vi "Plot Y-axis visibility.vi"(7 "Force update? (F)":bool, 8 "error in (no error)":errorcluster, 10 "top array":T1[](array[typedef]), 11 "Refs":T2) -> (0 "error out":errorcluster)   [LabVIEW 2021, in "RocketPlot.lvlib"]
uses:
  RocketPlot.lvlib
  TypeDefs/Plot UI references.ctl
  Classes/RocketPlotHandle/RocketPlotHandle.lvclass
  <userlib>/bjustice/TipStripOOPanel/Classes/TipPanelHandle/TipPanelHandle.lvclass
  TypeDefs/Plot top row.ctl
  Plot scale refnum to LUT name.vi
  FormatStringTime.vi
  Plot AxisFocus position.vi
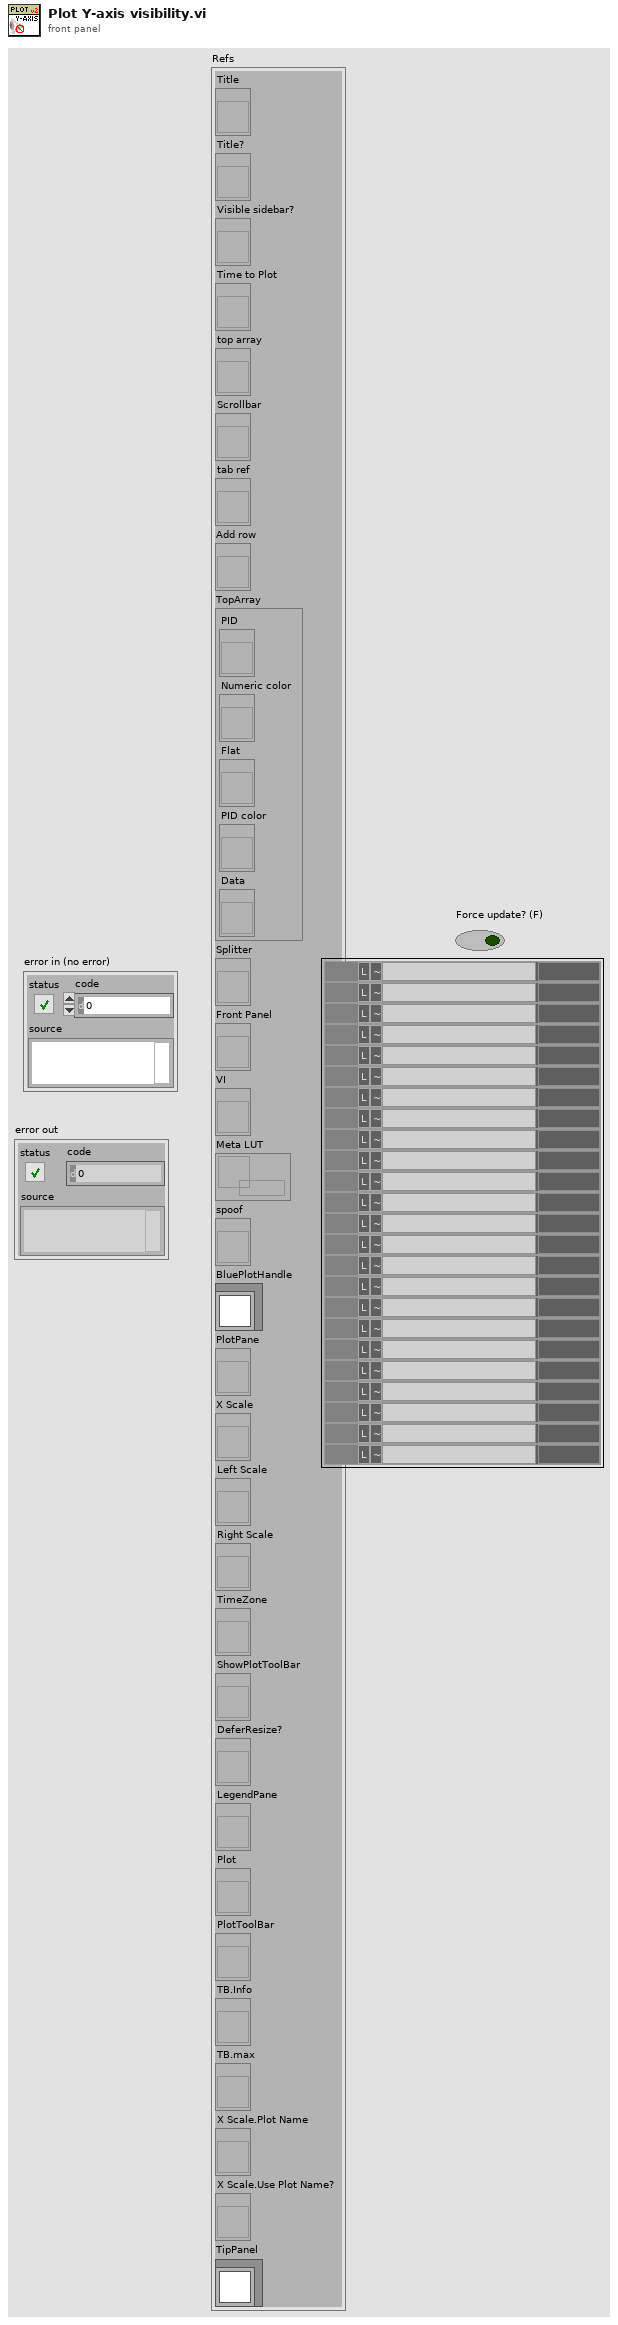
[diagram p1: front panel]
types:
  T1 = typedef "RocketPlot.lvlib/Plot top row.ctl" = cluster{"PID":string, "index":i32, "PID color":u32, "right axis?":bool, "Flatline?":bool, "Numeric color":u32, "Data":string, "Flat":string}
  T2 = typedef "RocketPlot.lvlib/Plot UI references.ctl" = cluster{"Title":refnum<vi>, "Title?":refnum<vi>, "Visible sidebar?":refnum<vi>, "Time to Plot":refnum<vi>, "top array":refnum<vi>, "Scrollbar":refnum<vi>, "tab ref":refnum<vi>, "Add row":refnum<vi>, "TopArray":cluster{"PID":refnum<vi>, "Numeric color":refnum<vi>, "Flat":refnum<vi>, "PID color":refnum<vi>, "Data":refnum<vi>}, "Splitter":refnum<vi>, "Front Panel":refnum<vi>, "VI":refnum<vi>, "Meta LUT":refnum<data-value>, "spoof":refnum<vi>, "BluePlotHandle":refnum<class "RocketPlotHandle.lvclass">, "PlotPane":refnum<vi>, "X Scale":refnum<vi>, "Left Scale":refnum<vi>, "Right Scale":refnum<vi>, "TimeZone":refnum<vi>, "ShowPlotToolBar":refnum<vi>, "DeferResize?":refnum<vi>, "LegendPane":refnum<vi>, "Plot":refnum<vi>, "PlotToolBar":refnum<vi>, "TB.Info":refnum<vi>, "TB.max":refnum<vi>, "X Scale.Plot Name":refnum<vi>, "X Scale.Use Plot Name?":refnum<vi>, "TipPanel":refnum<class "TipPanelHandle.lvclass">}
  T3 = typedef "TimeZone.ctl" = enum16{"UTC", "Local"}
  T4 = typedef "RocketPlot.lvlib/Plot scale meta JSON.ctl" = cluster{"Type":T5, "Grid Colors:Major Color":u32, "Grid Colors:Minor Color":u32, "Style":u8, "Tick Colors:Tick Color":u32, "Tick Colors:Minor Tick Color":u32, "Format String":string, "State":T6, "AxisFocus":refnum<vi>}
  T5 = typedef "RocketPlot.lvlib/Plot axis.ctl" = enum16{"x axis", "left axis", "right axis"}
  T6 = typedef "RocketPlot.lvlib/Plot scale meta state.ctl" = cluster{"Visible":bool, "Focus":bool, "Multi-Y":bool}
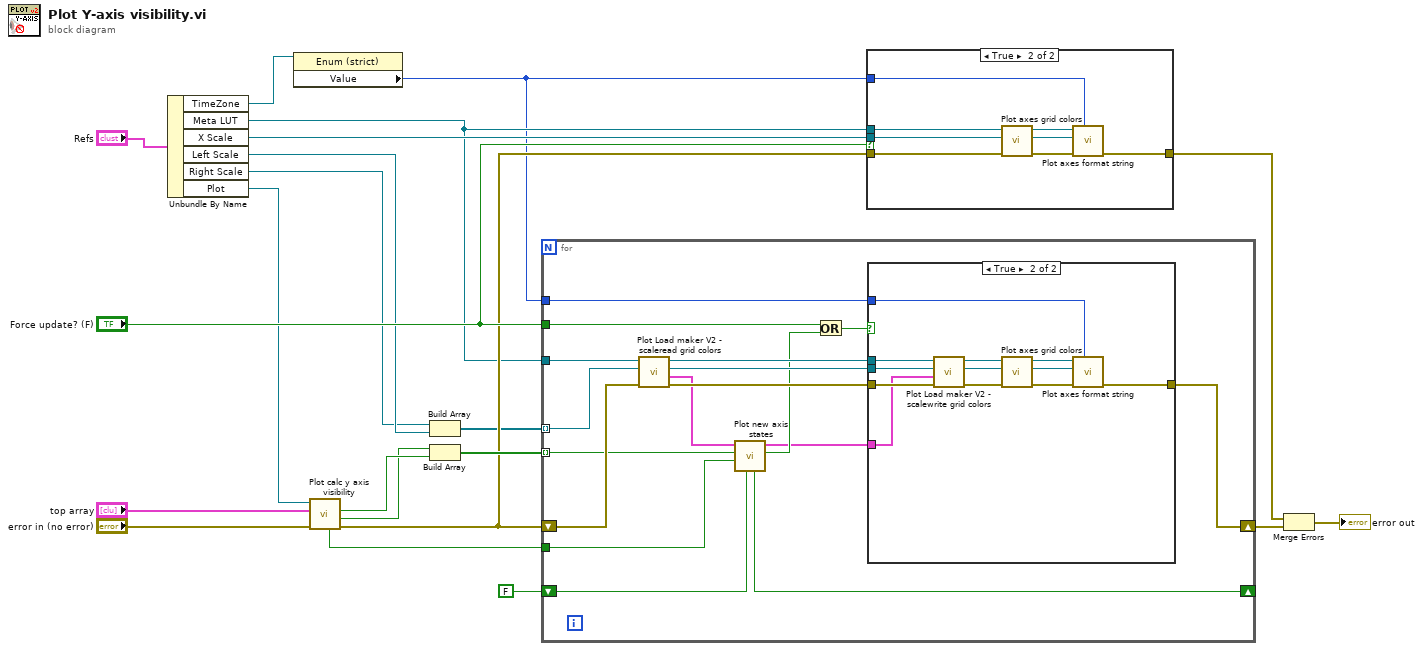
[diagram p0: block diagram]
diagram:
  n1 = Unbundle By Name("Refs") -> ("TimeZone"=w15:refnum<vi>, "Meta LUT"=w6:refnum<data-value>, "X Scale"=w8:refnum<vi>, "Left Scale"=w11:refnum<vi>, "Right Scale"=w10:refnum<vi>, "Plot"=w7:refnum<vi>)
  n2 = property class="Enum (strict)"(reference=w15) -> ("Value"=w5:T3)  [unwired: 1 in, 2 out]
  n3 = call "Plot calc y axis visibility.vi"("error in (no error)"="error in (no error)", "top array"="top array", "Plot"=w7) -> ("error out"=w14:errorcluster, "Right axis visible?"=w12:bool, "Left axis visible?"=w13:bool, "Multi-Y?"=w4:bool)  [unwired: 4 in, 1 out]
  n4 = Build Array(w10, w11) -> (w9:refnum<vi>[])
  n5 = Build Array(w12, w13) -> (w21:bool[])
  n6 = for {
    shift-right: [w38] -> w20
    shift-left: w14 -> [w32]
    tunnel: w21 -> [w26] mode=indexing
    tunnel: w6 -> [w37]
    tunnel: "Force update? (F)" -> [w30]
    tunnel: w9 -> [w33] mode=indexing
    tunnel: w5 -> [w31]
    tunnel: w4 -> [w25]
    shift-right: [w22] -> _
    shift-left: FALSE ("Multi-Y?") -> [w23]
    n7 = call "Plot Load maker V2 - scaleread grid colors.vi"("error in (no error)"=w32, "Scale reference"=w33, "Meta LUT"=w37) -> ("error out"=w34:errorcluster, "Scale LUT meta"=w28:T4, "Scale reference"=w36:refnum<vi>, "Meta LUT"=w35:refnum<data-value>)  [unwired: 5 in]
    n8 = call "Plot new axis states.vi"("GiveFocus?"=w23, "Multi-Y?"=w25, "Visible"=w26, "Scale LUT meta"=w28) -> ("state change?"=w27:bool, "Scale LUT meta"=w24:T4, "Multi-y & no-focus"=w22:bool)  [unwired: 5 in]
    n9 = Or(x=w30, y=w27) -> (x .or. y?=w29:bool)
    n10 = case shown="True" w29 {
      tunnel: [w39 w44] -> w38
      tunnel: w36 -> [_ w51]
      tunnel: w35 -> [_ w50]
      tunnel: w34 -> [w39 w49]
      tunnel: w31 -> [_ w40]
      tunnel: w24 -> [_ w41]
      frame False {
      }
      frame True {
        n11 = call "Plot Load maker V2 - scalewrite grid colors.vi"("error in (no error)"=w49, "Meta"=w41, "Scale reference"=w51, "Meta LUT"=w50) -> ("error out"=w47:errorcluster, "Scale reference"=w48:refnum<vi>, "Meta LUT"=w46:refnum<data-value>)  [unwired: 5 in]
        n12 = call "Plot axes grid colors.vi"("error in (no error)"=w47, "Scale reference"=w48, "Meta LUT"=w46) -> ("error out"=w45:errorcluster, "Scale reference"=w42:refnum<vi>, "Meta LUT"=w43:refnum<data-value>)  [unwired: 6 in]
        n13 = call "Plot axes format string.vi"("TimeZone"=w40, "error in (no error)"=w45, "Scale reference"=w42, "Meta LUT"=w43) -> ("error out"=w44:errorcluster)  [unwired: 6 in, 1 out]
      }
    }
  }
  n14 = case shown="True" "Force update? (F)" {
    tunnel: w6 -> [_ w54]
    tunnel: w14 -> [w52 w56]
    tunnel: [w52 w59] -> w19
    tunnel: w5 -> [_ w53]
    tunnel: w8 -> [_ w55]
    frame False {
    }
    frame True {
      n15 = call "Plot axes grid colors.vi"("error in (no error)"=w56, "Scale reference"=w55, "Meta LUT"=w54) -> ("error out"=w60:errorcluster, "Scale reference"=w58:refnum<vi>, "Meta LUT"=w57:refnum<data-value>)  [unwired: 6 in]
      n16 = call "Plot axes format string.vi"("TimeZone"=w53, "error in (no error)"=w60, "Scale reference"=w58, "Meta LUT"=w57) -> ("error out"=w59:errorcluster)  [unwired: 6 in, 1 out]
    }
  }
  n17 = Merge Errors(w19, w20) -> (→"error out":errorcluster)
